vi "Facade.vi"(0 "Data In":T5, 2 "Display State In":T3, 3 "Container State":T4) -> (6 "Data Out":T5, 7 "Display State Out":T3, 8 "Action":T2)   [LabVIEW 2020, in "Gate.xctl"]
uses:
  Gate.xctl
  Data.ctl
  Classes/Gate/Gate.lvclass
  <vilib>/_xctls/Container State.ctl
  State.ctl
  <vilib>/_xctls/Action.ctl
  Utility VIs/Controls/KCheckbox/KCheckbox.xctl
  Classes/Gate/Gate.lvclass/Gate.ctl
  Classes/Gate/Shape.ctl
  Classes/Gate/Read Shape.vi
  Classes/Gate/Read Delay (ms).vi
  Classes/Gate/Read Duration (ms).vi
  Classes/Gate/Read Repeat.vi
  Classes/Gate/Read Rate (Hz).vi
  Classes/Gate/Read Trepeat (ms).vi
  Classes/Gate/Write Shape.vi
  Classes/Gate/Write Delay (ms).vi
  Classes/Gate/Write Duration (ms).vi
  Classes/Gate/Write Ramp (ms).vi
  Classes/Gate/Write Down (ms).vi
  Classes/Gate/Write Asymmetric.vi
  Classes/Gate/Write Repeat.vi
  Classes/Gate/Write Rate (Hz).vi
  Classes/Gate/Write Trepeat (ms).vi
  Classes/Gate/Read Ramp (ms).vi
  Classes/Gate/Read Down (ms).vi
  Classes/Gate/Read Asymmetric.vi
  <vilib>/_xctls/XControlSupport.lvlib
panel:
  in  "Delta (dB)":dbl
  in  "Invert":bool(xcontrol) caption="Repeat"
  in  "Delay (ms)":dbl
  in  "Shape":T1(ring)
  in  "Ramp (ms)":string
  in  "Duration (ms)":dbl
  in  "for":dbl caption="ms"
  in  "at":dbl caption="Hz"
  in  "Repeat":bool(xcontrol)
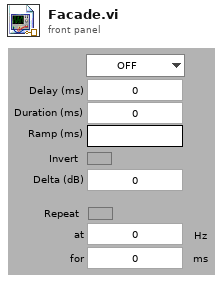
[diagram p1: front panel]
types:
  T1 = enum16{"OFF", "Rectangle", "Sine-squared", "Trapezoid"}
  T2 = typedef "XControlSupport.lvlib/Action.ctl" = cluster{"Data Changed?":bool, "State Changed?":bool, "Action Name":string}
  T3 = typedef "Gate.xctl/State.ctl" = cluster{"Numeric":dbl}
  T4 = typedef "XControlSupport.lvlib/Container State.ctl" = cluster{"Indicator?":bool, "Run Mode?":bool, " Refnum":refnum<vi>}
  T5 = typedef "Gate.xctl/Data.ctl" = refnum<class "Gate.lvclass">
  T6 = typedef "Gate.lvclass/Shape.ctl" = enum16{"OFF", "Rectangle", "Sine-squared", "Trapezoid"}
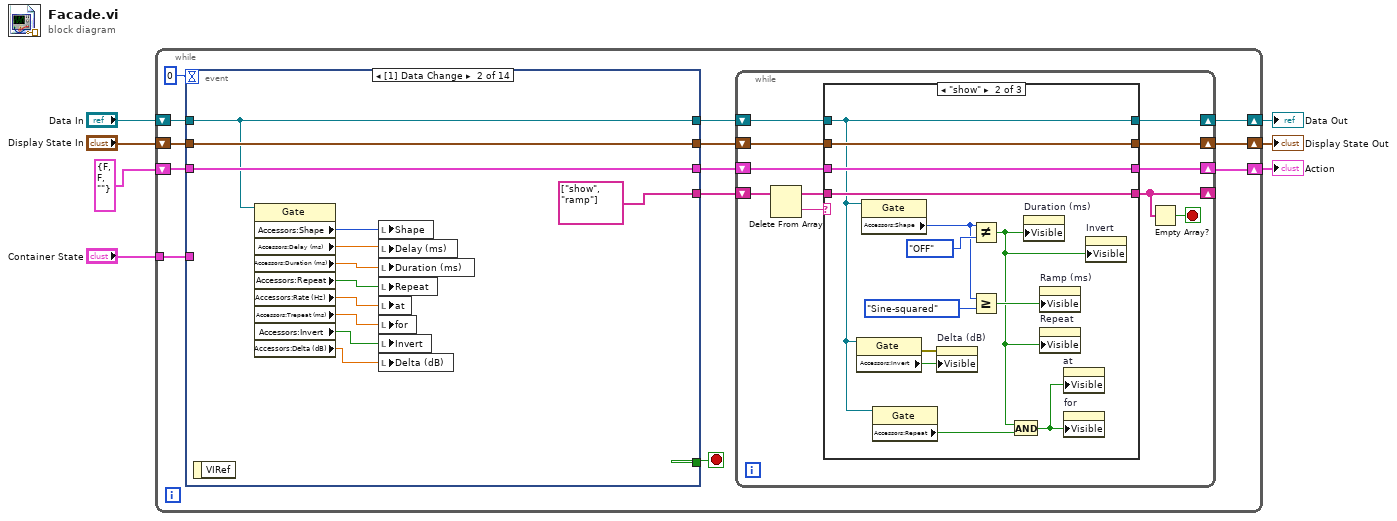
[diagram p0: block diagram]
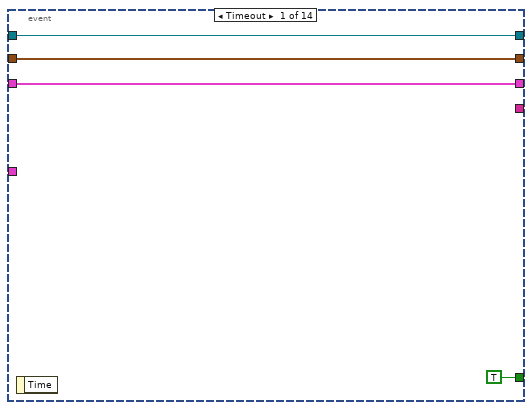
[diagram p2: hidden frame]
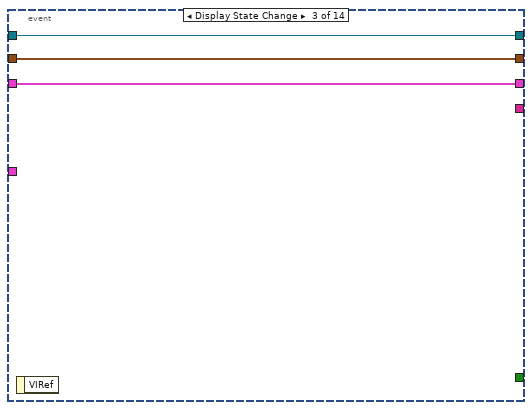
[diagram p3: hidden frame]
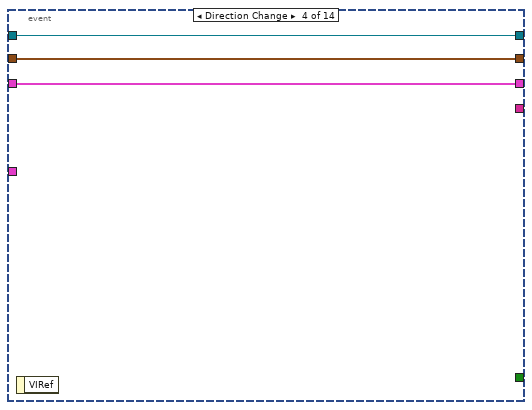
[diagram p4: hidden frame]
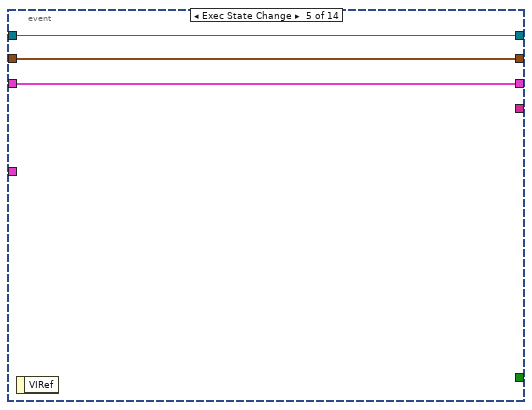
[diagram p5: hidden frame]
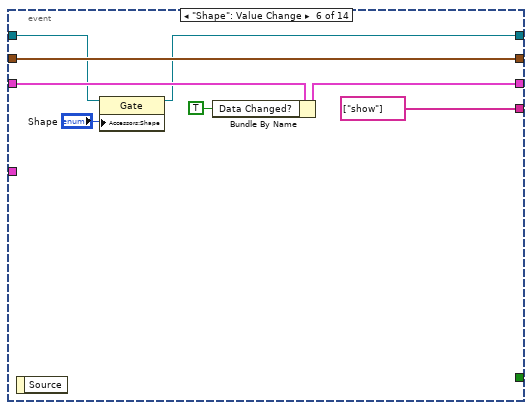
[diagram p6: hidden frame]
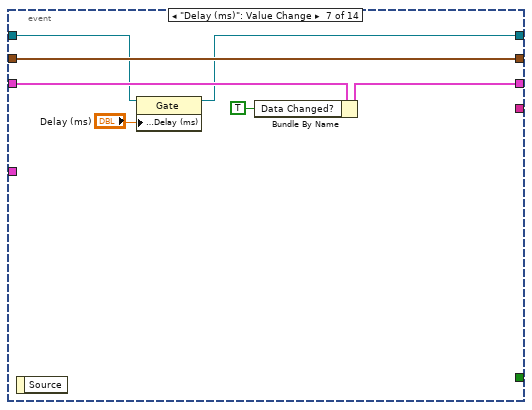
[diagram p7: hidden frame]
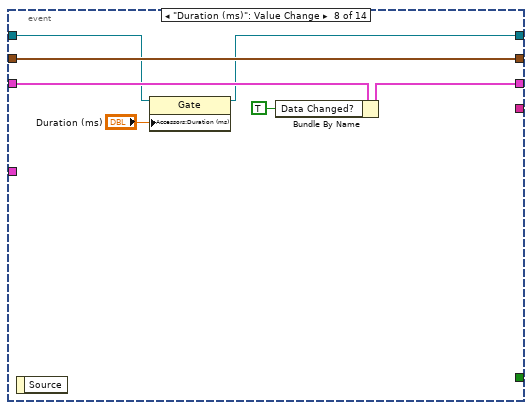
[diagram p8: hidden frame]
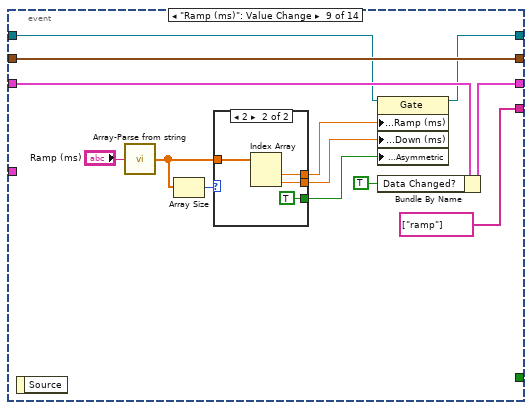
[diagram p9: hidden frame]
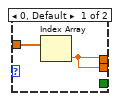
[diagram p10: hidden frame]
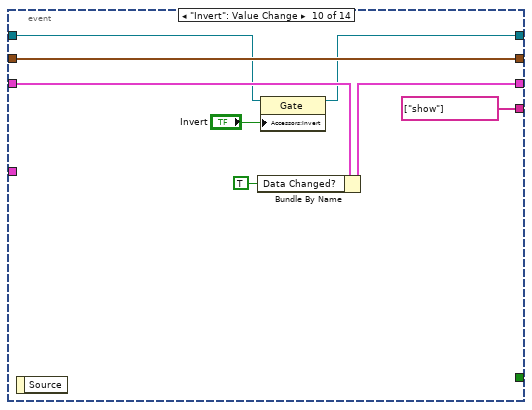
[diagram p11: hidden frame]
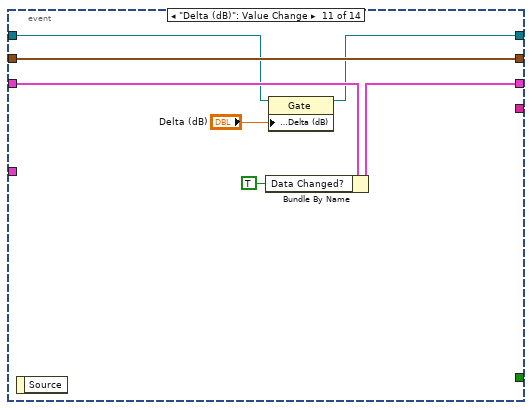
[diagram p12: hidden frame]
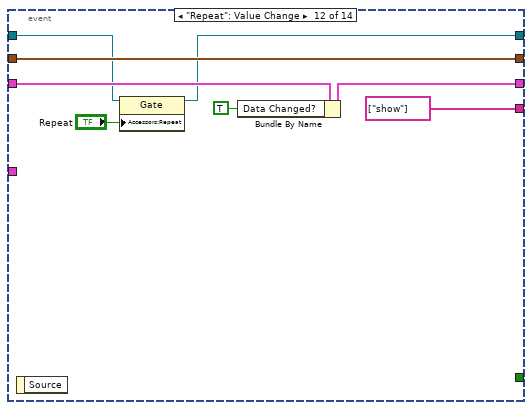
[diagram p13: hidden frame]
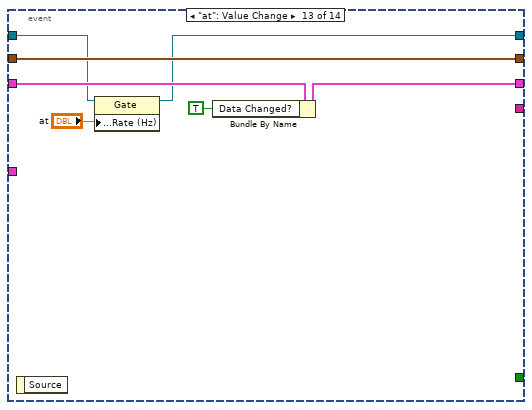
[diagram p14: hidden frame]
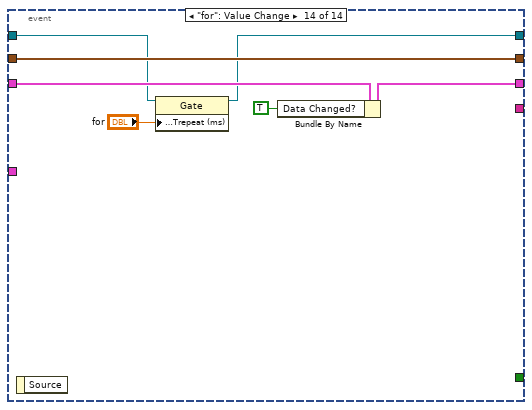
[diagram p15: hidden frame]
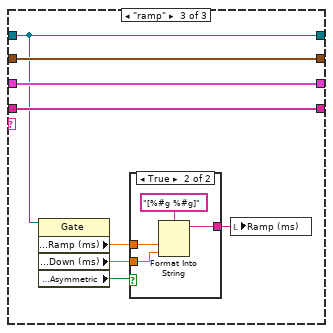
[diagram p17: hidden frame]
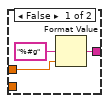
[diagram p18: hidden frame]
diagram:
  n1 = while {
    shift-right: [w12] -> w4
    shift-left: "Display State In" -> [w20]
    tunnel: "Container State" -> [w17]
    shift-right: [w14] -> w7
    shift-left: "Data In" -> [w16]
    shift-right: [w10] -> w2
    shift-left: T2 {"Data Changed?"=FALSE, "State Changed?"=FALSE, "Action Name"=""} ("Action") -> [w15]
    stop <- w19 stop-if-true
    n2 = event shown="[1] Data Change" {
      selector: _ -> [_ _ _ _ _ _ _ _ _ _ _ _ _ _]
      dyn-events: _ -> [_ _ _ _ _ _ _ _ _ _ _ _ _ _]
      timeout: 0 -> [_ _ _ _ _ _ _ _ _ _ _ _ _ _]
      tunnel: w20 -> [w22 w36 w37 w42 w45 w53 w60 w67 w80 w94 w101 w109 w116 w123]
      tunnel: [w22 w36 w37 w42 w45 w53 w60 w67 w80 w94 w101 w109 w116 w123] -> w11
      tunnel: [TRUE _ _ _ _ _ _ _ _ _ _ _ _ _] -> w19
      tunnel: w17 -> [_ _ _ _ _ _ _ _ _ _ _ _ _ _]
      tunnel: w16 -> [w21 w34 w38 w41 w44 w50 w58 w65 w78 w92 w99 w106 w114 w121]
      tunnel: [w21 w34 w38 w41 w44 w49 w57 w64 w77 w91 w98 w105 w113 w120] -> w13
      tunnel: [w23 w35 w39 w40 w43 w48 w56 w63 w76 w90 w97 w104 w112 w119] -> w9
      tunnel: w15 -> [w23 w35 w39 w40 w43 w52 w59 w66 w79 w93 w100 w108 w115 w122]
      tunnel: [_ string[] ["show", "ramp"] _ _ _ string[] ["show"] _ _ string[] ["ramp"] string[] ["show"] _ string[] ["show"] _ _] -> w8
      event Timeout {
        n3 = event-data() -> ()  [unwired: 1 in, 1 out]
      }
      event Data Change {
        n4 = event-data() -> ()  [unwired: 1 in, 1 out]
        n5 = property class="Gate"(reference=w34) -> ("Accessors:Shape"=w33:T6, "Accessors:Delay (ms)"=w31:dbl, "Accessors:Duration (ms)"=w30:dbl, "Accessors:Repeat"=w29:bool, "Accessors:Rate (Hz)"=w28:dbl, "Accessors:Trepeat (ms)"=w27:dbl, "Accessors:Invert"=w26:bool, "Accessors:Delta (dB)"=w25:dbl)  [unwired: 1 in, 2 out]
        n6 = local write "Shape"(w33) -> ()
        n7 = local write "Delay (ms)"(w31) -> ()
        n8 = local write "Duration (ms)"(w30) -> ()
        n9 = local write "Repeat"(w29) -> ()
        n10 = local write "at"(w28) -> ()
        n11 = local write "for"(w27) -> ()
        n12 = local write "Invert"(w26) -> ()
        n13 = local write "Delta (dB)"(w25) -> ()
      }
      event Display State Change {
        n14 = event-data() -> ()  [unwired: 1 in, 1 out]
      }
      event Direction Change {
        n15 = event-data() -> ()  [unwired: 1 in, 1 out]
      }
      event Exec State Change {
        n16 = event-data() -> ()  [unwired: 1 in, 1 out]
      }
      event "Shape": Value Change {
        n17 = event-data() -> ()  [unwired: 1 in, 1 out]
        n18 = property class="Gate"(reference=w50, "Accessors:Shape"="Shape") -> (reference out=w49:T5)  [unwired: 1 in, 1 out]
        n19 = Bundle By Name(cluster=w52, "Data Changed?"=TRUE) -> (w48:T2)
      }
      event "Delay (ms)": Value Change {
        n20 = event-data() -> ()  [unwired: 1 in, 1 out]
        n21 = property class="Gate"(reference=w58, "Accessors:Delay (ms)"="Delay (ms)") -> (reference out=w57:T5)  [unwired: 1 in, 1 out]
        n22 = Bundle By Name(cluster=w59, "Data Changed?"=TRUE) -> (w56:T2)
      }
      event "Duration (ms)": Value Change {
        n23 = event-data() -> ()  [unwired: 1 in, 1 out]
        n24 = property class="Gate"(reference=w65, "Accessors:Duration (ms)"="Duration (ms)") -> (reference out=w64:T5)  [unwired: 1 in, 1 out]
        n25 = Bundle By Name(cluster=w66, "Data Changed?"=TRUE) -> (w63:T2)
      }
      event "Ramp (ms)": Value Change {
        n26 = event-data() -> ()  [unwired: 1 in, 1 out]
        n27 = call "Array-Parse from string.vi"("String"="Ramp (ms)") -> ("Array"=w72:dbl[])  [unwired: 13 in, 1 out]
        n28 = Array Size(array=w72) -> (size(s)=w73:i32)
        n29 = case shown="2" w73 {
          tunnel: w72 -> [w82 w86]
          tunnel: [w81 w85] -> w71
          tunnel: [w81 w84] -> w70
          tunnel: [_ TRUE] -> w69
          frame 0, Default {
            n30 = Index Array(array=w82) -> (element=w81:dbl)  [unwired: 1 in]
          }
          frame 2 {
            n31 = Index Array(array=w86) -> (element #1=w85:dbl, element #2=w84:dbl)  [unwired: 2 in]
          }
        }
        n32 = property class="Gate"(reference=w78, "Accessors:Ramp (ms)"=w71, "Accessors:Down (ms)"=w70, "Accessors:Asymmetric"=w69) -> (reference out=w77:T5)  [unwired: 1 in, 1 out]
        n33 = Bundle By Name(cluster=w79, "Data Changed?"=TRUE) -> (w76:T2)
      }
      event "Invert": Value Change {
        n34 = event-data() -> ()  [unwired: 1 in, 1 out]
        n35 = Bundle By Name(cluster=w93, "Data Changed?"=TRUE) -> (w90:T2)
        n36 = property class="Gate"(reference=w92, "Accessors:Invert"="Invert") -> (reference out=w91:T5)  [unwired: 1 in, 1 out]
      }
      event "Delta (dB)": Value Change {
        n37 = event-data() -> ()  [unwired: 1 in, 1 out]
        n38 = Bundle By Name(cluster=w100, "Data Changed?"=TRUE) -> (w97:T2)
        n39 = property class="Gate"(reference=w99, "Accessors:Delta (dB)"="Delta (dB)") -> (reference out=w98:T5)  [unwired: 1 in, 1 out]
      }
      event "Repeat": Value Change {
        n40 = event-data() -> ()  [unwired: 1 in, 1 out]
        n41 = property class="Gate"(reference=w106, "Accessors:Repeat"="Repeat") -> (reference out=w105:T5)  [unwired: 1 in, 1 out]
        n42 = Bundle By Name(cluster=w108, "Data Changed?"=TRUE) -> (w104:T2)
      }
      event "at": Value Change {
        n43 = event-data() -> ()  [unwired: 1 in, 1 out]
        n44 = property class="Gate"(reference=w114, "Accessors:Rate (Hz)"="at") -> (reference out=w113:T5)  [unwired: 1 in, 1 out]
        n45 = Bundle By Name(cluster=w115, "Data Changed?"=TRUE) -> (w112:T2)
      }
      event "for": Value Change {
        n46 = event-data() -> ()  [unwired: 1 in, 1 out]
        n47 = property class="Gate"(reference=w121, "Accessors:Trepeat (ms)"="for") -> (reference out=w120:T5)  [unwired: 1 in, 1 out]
        n48 = Bundle By Name(cluster=w122, "Data Changed?"=TRUE) -> (w119:T2)
      }
    }
    n49 = while {
      shift-right: [w131] -> _
      shift-left: w8 -> [w134]
      shift-right: [w129] -> w14
      shift-left: w13 -> [w128]
      shift-right: [w127] -> w12
      shift-left: w11 -> [w126]
      shift-right: [w125] -> w10
      shift-left: w9 -> [w124]
      stop <- w130 stop-if-true
      n50 = Delete From Array(array=w134) -> (deleted portion=w132:string, array with subset deleted=w133:string[])  [unwired: 2 in]
      n51 = case shown="\"show\"" w132 {
        tunnel: w133 -> [w138 w151 w159]
        tunnel: [w138 w151 w159] -> w131
        tunnel: [w137 w141 w152] -> w129
        tunnel: w128 -> [w137 w141 w152]
        tunnel: [w136 w150 w158] -> w127
        tunnel: w126 -> [w136 w150 w158]
        tunnel: [w135 w149 w157] -> w125
        tunnel: w124 -> [w135 w149 w157]
        frame "", Default {
        }
        frame "show" {
          n52 = property class="Gate"(reference=w141) -> (error out=w140:errorcluster, "Accessors:Invert"=w139:bool)  [unwired: 1 in, 1 out]
          n53 = property class="Gate"(reference=w141) -> ("Accessors:Shape"=w145:T6)  [unwired: 1 in, 2 out]
          n54 = property class="Gate"(reference=w141) -> ("Accessors:Repeat"=w148:bool)  [unwired: 1 in, 2 out]
          n55 = property on="Delta (dB)" class="DigNum (strict)"(error in=w140, "Visible"=w139) -> ()  [unwired: 1 in, 2 out]
          n56 = Not Equal?(x=w145, y=Shape."OFF") -> (x != y?=w142:bool)
          n57 = Greater Or Equal?(x=w145, y=Shape."Sine-squared") -> (x >= y?=w143:bool)
          n58 = And(x=w142, y=w148) -> (x .and. y?=w147:bool)
          n59 = property on="Duration (ms)" class="DigNum (strict)"("Visible"=w142) -> ()  [unwired: 2 in, 2 out]
          n60 = property on="Ramp (ms)" class="Str"("Visible"=w143) -> ()  [unwired: 2 in, 2 out]
          n61 = property on="Repeat" class="KCheckbox (strict)"("Visible"=w142) -> ()  [unwired: 2 in, 2 out]
          n62 = property on="at" class="DigNum (strict)"("Visible"=w147) -> ()  [unwired: 2 in, 2 out]
          n63 = property on="for" class="DigNum (strict)"("Visible"=w147) -> ()  [unwired: 2 in, 2 out]
          n64 = property on="Invert" class="KCheckbox (strict)"("Visible"=w142) -> ()  [unwired: 2 in, 2 out]
        }
        frame "ramp" {
          n65 = property class="Gate"(reference=w152) -> ("Accessors:Ramp (ms)"=w155:dbl, "Accessors:Down (ms)"=w154:dbl, "Accessors:Asymmetric"=w153:bool)  [unwired: 1 in, 2 out]
          n66 = case shown="True" w153 {
            tunnel: w155 -> [w162 w165]
            tunnel: w154 -> [_ w163]
            tunnel: [w161 w164] -> w156
            frame False {
              n67 = Format Value(format string="%#g", value (0)=w162) -> (output string=w161:string)  [unwired: 1 in]
            }
            frame True {
              n68 = Format Into String(format string="[%#g %#g]", w165, w163) -> (resulting string=w164:string)  [unwired: 2 in, 1 out]
            }
          }
          n69 = local write "Ramp (ms)"(w156) -> ()
        }
      }
      n70 = Empty Array?(array=w131) -> (empty?=w130:bool)
    }
  }
  "Display State Out" <- w4
  "Data Out" <- w7
  "Action" <- w2
